vi "Load Simulation AVI.vi"(8 "error in (no error)":errorcluster) -> (0 "error out":errorcluster, 3 "Words per image":u32)   [LabVIEW 2013]
uses:
  Globals/Simulation Settings Global.vi
  <vilib>/rvi/interface/nirviMethod/nirviMethod.xnode
  Image Acquisition/Image Acquisition Settings FG Enum.ctl
  <vilib>/rvi/interface/nirviReadWriteControl/nirviReadWriteControl.xnode
  FGs/FPGA_Reference.ctl
  <vilib>/rvi/errors/niLvFpgaMergeErrorWithErrorCode.vi
  FPGA Bitfiles/WBA256Sectors_FPGATarget.lvbitx
  NiFpgaLv.dll
  <vilib>/Utility/error.llb/Error Cluster From Error Code.vi
  <vilib>/rvi/errors/niLvFpgaAdjustHostInterfaceError.vi
  <vilib>/FPGAPlugInAG/PCIe-1473R-LX110/niLvFpga_ConfigureFifo_PCIe-1473R-LX110.vi
  <vilib>/FPGAPlugInAG/PCIe-1473R-LX110/niLvFpga_StartFifo_PCIe-1473R-LX110.vi
  <vilib>/FPGAPlugInAG/PCIe-1473R-LX110/niLvFpga_WriteFifo_PCIe-1473R-LX110.vi
panel:
  out "Enum":T1(ring)
  out "Requested Depth":u32
  out "Actual Depth":u32
  out "Bytes per image":u32
  out "Number of Frames":u32
  out "Frame Data":T2
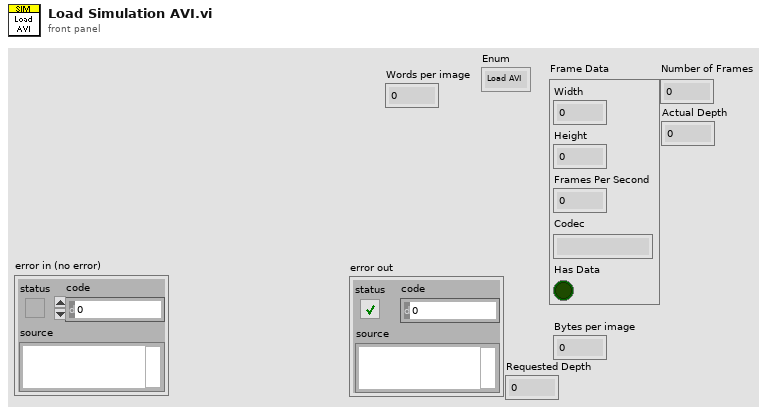
[diagram p1: front panel]
types:
  T1 = enum16{"Load AVI", "Configure FIFOs", "Convert Data to 10 Tap", "Close AVI"}
  T2 = cluster{"Width":u32, "Height":u32, "Frames Per Second":u32, "Codec":string, "Has Data":bool}
  T3 = typedef "Image Acquisition Settings FG Enum.ctl" = enum16{"Read", "Write"}
  T4 = typedef "Simulation Settings Cluster.ctl" = cluster{"Sim Enabled?":bool, "Sim Path":path}
  T5 = typedef "IMAQ AVI2 Refnum.ctl" = refnum<k20>
  T6 = typedef "FPGA_Reference.ctl" = refnum<k20>
  T7 = typedef "Acquisition Settings Cluster.ctl" = cluster{"Image Width":u32, "Image Height":u32, "Frames To Acquire":u32, "Signal Mapping":enum8{"Standard", "Basler 10-tap", "Vosskühler 10-tap"}, "DMA Buffer Size\n(In Images)":u32}
  T8 = typedef "IMAQ Image.ctl" = refnum<image>
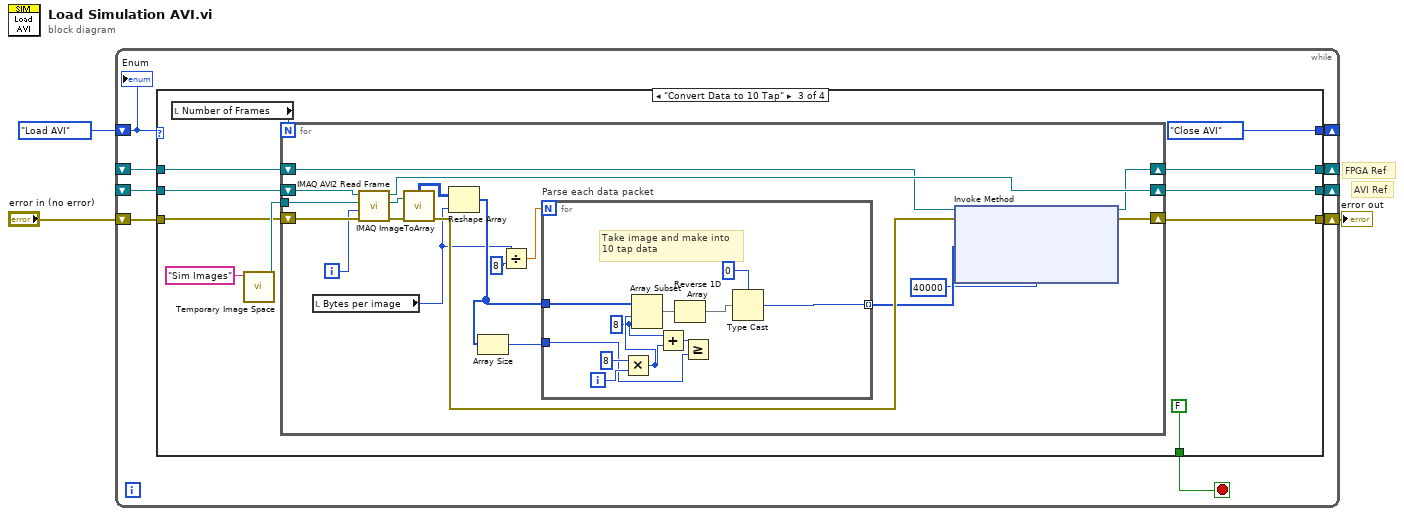
[diagram p0: block diagram]
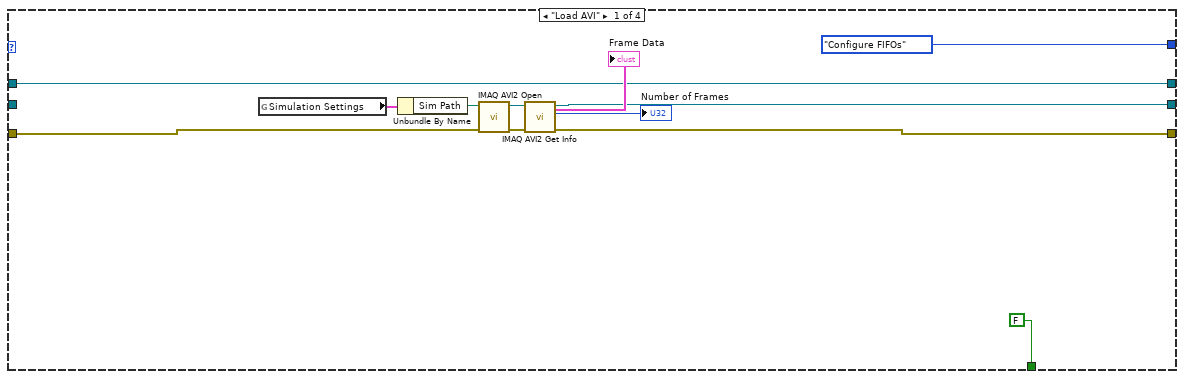
[diagram p2: hidden frame]
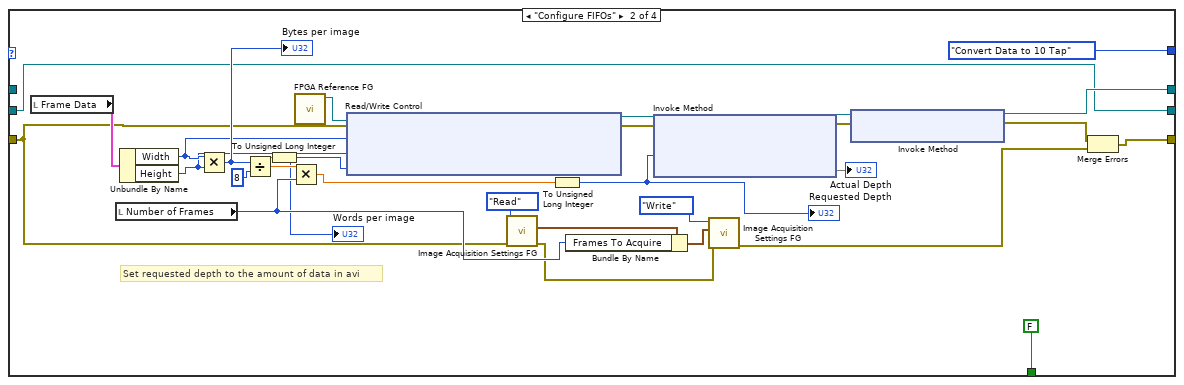
[diagram p3: hidden frame]
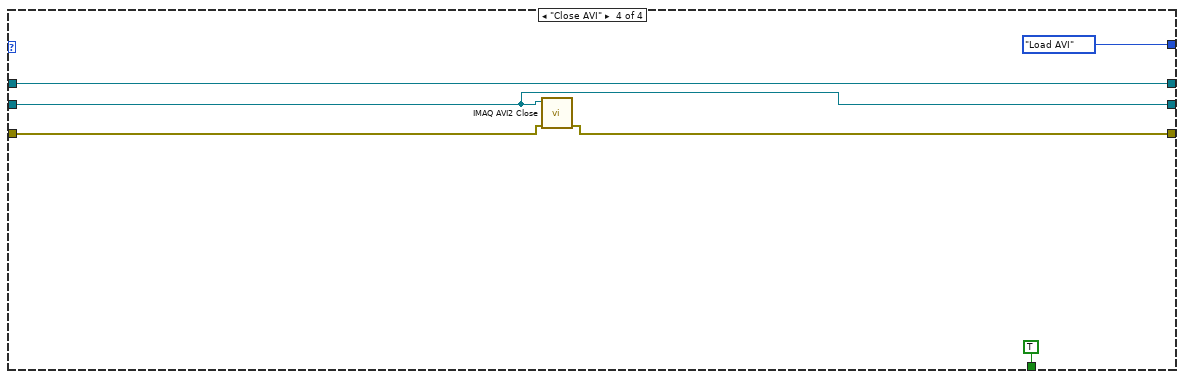
[diagram p4: hidden frame]
diagram:
  # "AVI Ref"
  # "FPGA Ref"
  n1 = while {
    shift-right: [w8] -> _
    shift-left: T1."Load AVI" -> [w12]
    shift-right: [w11] -> _
    shift-left: _ -> [w5]
    shift-right: [w10] -> w1
    shift-left: "error in (no error)" -> [w9]
    shift-right: [w6] -> _
    shift-left: _ -> [w4]
    stop <- w7 stop-if-true
    n2 = case shown="\"Convert Data to 10 Tap\"" w12 {
      tunnel: w9 -> [w20 w33 w59 w98]
      tunnel: [w18 w47 w55 w96] -> w11
      tunnel: [w17 w40 w54 w97] -> w10
      tunnel: [T1."Configure FIFOs" T1."Convert Data to 10 Tap" T1."Close AVI" T1."Load AVI"] -> w8
      tunnel: [FALSE FALSE FALSE TRUE] -> w7
      tunnel: [w13 w50 w56 w99] -> w6
      tunnel: w5 -> [_ w47 w58 w96]
      tunnel: w4 -> [w13 _ w57 w99]
      frame "Load AVI" {
        n3 = global read "Simulation Settings Global.vi" "Simulation Settings"() -> (w21:T4)
        n4 = Unbundle By Name(w21) -> ("Sim Path"=w22:path)
        n5 = call "IMAQ AVI2 Open"("error in (no error)"=w20, "AVI File Path"=w22) -> ("error out"=w23:errorcluster, "AVI Refnum"=w24:T5)  [unwired: 8 in]
        n6 = call "IMAQ AVI2 Get Info"("error in (no error)"=w23, "AVI Refnum"=w24) -> ("error out"=w17:errorcluster, "Number of Frames"=→"Number of Frames":u32, "AVI Refnum (duplicate)"=w18:T5, "Frame Data"=→"Frame Data":T2)  [unwired: 5 in, 1 out]
      }
      frame "Configure FIFOs" {
        # "Set requested depth to the amount of data in avi"
        n7 = local read "Frame Data"() -> (w51:T2)
        n8 = local read "Number of Frames"() -> (w42:u32)
        n9 = Unbundle By Name(w51) -> ("Width"=w32:u32, "Height"=w31:u32)
        n10 = Multiply(x=w32, y=w31) -> (x*y=w53:u32)
        "Bytes per image" <- w53
        n11 = Divide(x=w53, y=u32 8) -> (x/y=w30:dbl)
        n12 = To Unsigned Long Integer(number=w30) -> (unsigned 32bit integer=w29:u32)
        "Words per image" <- w29
        n13 = Multiply(x=w30, y=w42) -> (x*y=w27:dbl)
        n14 = call "FPGA Reference FG.vi"() -> ("FPGA VI Reference Out"=w35:T6)  [unwired: 11 in]
        n15 = xnode "Read/Write Control"("FPGA VI Reference In"=w35, "error in"=w33, "X Resolution"=w32, "Y Resolution"=w31, "Words per image"=w29) -> ("FPGA VI Reference Out"=w34:T6, "error out"=w25:errorcluster)
        n16 = call "Image Acquisition Settings FG.vi"("error in (no error)"=w33, "Operation"=Image_Acquisition_Settings_FG_Enum."Read") -> ("error out"=w41:errorcluster, "Acquisition Settings Out"=w45:T7)  [unwired: 8 in]
        n17 = To Unsigned Long Integer(number=w27) -> (unsigned 32bit integer=w28:u32)
        "Requested Depth" <- w28
        n18 = Bundle By Name(cluster=w45, "Frames To Acquire"=w42) -> (w44:T7)
        n19 = xnode "Invoke Method"("FPGA VI Reference In"=w34, "error in"=w25, "Requested Depth"=w28) -> ("FPGA VI Reference Out"=w36:T6, "error out"=w37:errorcluster, "Actual Depth"=→"Actual Depth")
        n20 = call "Image Acquisition Settings FG.vi"("error in (no error)"=w41, "Acquisition Settings In"=w44, "Operation"=Image_Acquisition_Settings_FG_Enum."Write") -> ("error out"=w38:errorcluster)  [unwired: 7 in, 1 out]
        n21 = xnode "Invoke Method"("FPGA VI Reference In"=w36, "error in"=w37) -> ("FPGA VI Reference Out"=w50:T6, "error out"=w39:errorcluster)
        n22 = Merge Errors(w39, w38) -> (w40:errorcluster)
      }
      frame "Convert Data to 10 Tap" {
        n23 = local read "Number of Frames"() -> (w63:u32)
        n24 = call "Temporary Image Space.vi"("Image Name"="Sim Images") -> ("Image Out"=w60:T8)  [unwired: 10 in]
        n25 = for {
          N: w63 -> [_]
          tunnel: w60 -> [w83]
          shift-right: [w71] -> w54
          shift-left: w59 -> [w82]
          shift-right: [w73] -> w55
          shift-left: w58 -> [w79]
          shift-right: [w70] -> w56
          shift-left: w57 -> [w72]
          i -> [w78]
          n26 = local read "Bytes per image"() -> (w68:u32)
          n27 = call "IMAQ AVI2 Read Frame"("error in (no error)"=w82, "Frame Number"=w78, "Image"=w83, "AVI Refnum"=w79) -> ("error out"=w81:errorcluster, "Image Out"=w80:T8, "AVI Refnum (duplicate)"=w73:T5)  [unwired: 5 in]
          n28 = call "IMAQ ImageToArray"("error in (no error)"=w81, "Image"=w80) -> ("error out"=w74:errorcluster, "Image Pixels (U8)"=w77:u8[][])  [unwired: 2 in, 3 out]
          n29 = Reshape Array(w77, w68) -> (w76:u8[])
          n30 = Array Size(array=w76) -> (size(s)=w75:i32)
          n31 = Divide(x=w68, y=u32 8) -> (x/y=w66:dbl)
          n32 = for "Parse each data packet" {
            N: w66 -> [_]
            tunnel: w75 -> [w88]
            tunnel: w76 -> [w92]
            tunnel: [w85] -> w69 mode=indexing
            i -> [w94]
            w90 = 8 ("length")
            # "Take image and make into\n10 tap data"
            n33 = Multiply(x=8, y=w94) -> (x*y=w91:i32)
            n34 = Array Subset(array=w92, index=w91, length=w90) -> (w87:u8[])
            n35 = Add(x=w90, y=w91) -> (x+y=w89:i32)
            n36 = Reverse 1D Array(array=w87) -> (reversed array=w84:u8[])
            n37 = Greater Or Equal?(x=w89, y=w88) -> ()  [unwired: 1 out]
            n38 = Type Cast(type=u64 0, x=w84) -> (*(type *) &x=w85:u64)
          }
          n39 = xnode "Invoke Method"("FPGA VI Reference In"=w72, "error in"=w74, "Data"=w69, "Timeout (ms)"=40000) -> ("FPGA VI Reference Out"=w70:T6, "error out"=w71:errorcluster)  [unwired: 1 out]
        }
      }
      frame "Close AVI" {
        n40 = call "IMAQ AVI2 Close"("error in (no error)"=w98, "AVI Refnum"=w96) -> ("error out"=w97:errorcluster)  [unwired: 9 in]
      }
    }
    "Enum" <- w12
  }
  "error out" <- w1
